vi "SliderAndBarTest.vi"(0 "Vertical Pointer Slide Control":dbl(slide) scale=0.0..10.0, 1 "Vertical Progress Bar Control":i32(slide) scale=0.0..100.0, 2 "Vertical Graduated Bar Control":u8(slide) scale=0.0..100.0, 3 "Horizontal Fill Slide Control":dbl(slide) scale=0.0..10.0, 4 "Horizontal Pointer Slide Control":dbl(slide) scale=0.0..10.0, 5 "Horizontal Progress Bar Control":u8(slide) scale=0.0..100.0, 6 "Vertical Fill Slide Control":dbl(slide) scale=0.0..10.0, 7 "Horizontal Graduated Bar Control":u8(slide) scale=0.0..100.0, 8 "Number To Add With":i32) -> (12 "Vertical Fill Slide Indicator":dbl(slide) scale=0.0..10.0, 13 "Horizontal Graduated Bar Indicator":u8(slide) scale=0.0..100.0, 14 "Vertical Pointer Slide Indicator":dbl(slide) scale=0.0..10.0, 15 "Vertical Progress Bar Indicator":i32(slide) scale=0.0..100.0, 16 "Vertical Graduated Bar Indicator":u8(slide) scale=0.0..100.0, 17 "Horizontal Fill Slide Indicator":dbl(slide) scale=0.0..10.0, 18 "Horizontal Pointer Slide Indicator":dbl(slide) scale=0.0..10.0, 19 "Horizontal Progress Bar Indicator":u8(slide) scale=0.0..100.0)   [LabVIEW 2012]
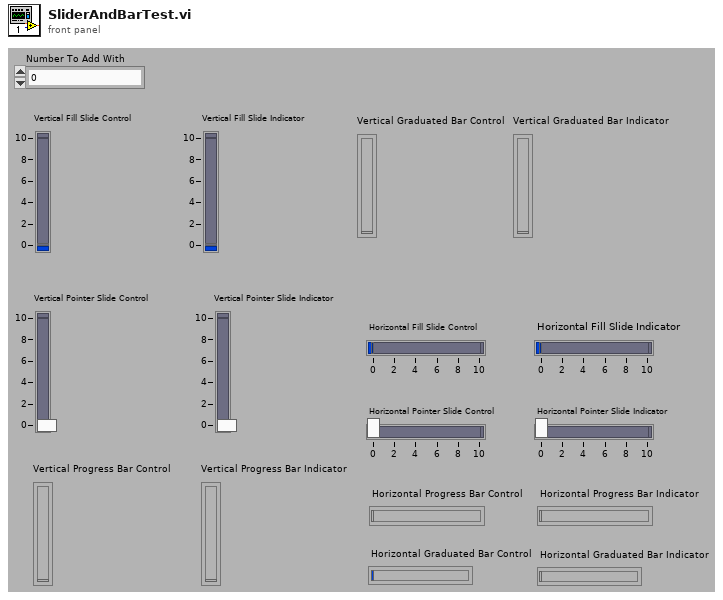
[diagram p1: front panel]
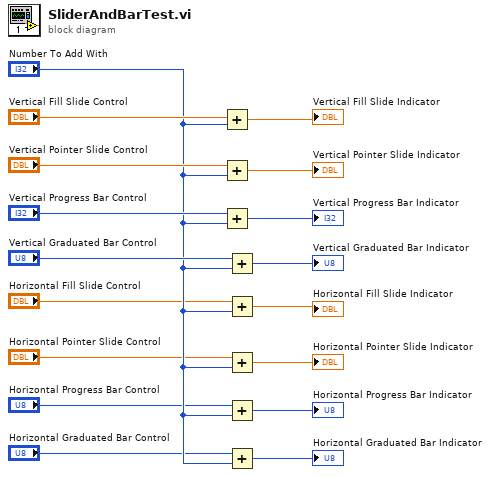
[diagram p0: block diagram]
diagram:
  n1 = Add(x="Vertical Fill Slide Control", y="Number To Add With") -> (x+y=→"Vertical Fill Slide Indicator":dbl)
  n2 = Add(x="Vertical Pointer Slide Control", y="Number To Add With") -> (x+y=→"Vertical Pointer Slide Indicator":dbl)
  n3 = Add(x="Vertical Progress Bar Control", y="Number To Add With") -> (x+y=→"Vertical Progress Bar Indicator":i32)
  n4 = Add(x="Vertical Graduated Bar Control", y="Number To Add With") -> (x+y=→"Vertical Graduated Bar Indicator":i32)
  n5 = Add(x="Horizontal Fill Slide Control", y="Number To Add With") -> (x+y=→"Horizontal Fill Slide Indicator":dbl)
  n6 = Add(x="Horizontal Pointer Slide Control", y="Number To Add With") -> (x+y=→"Horizontal Pointer Slide Indicator":dbl)
  n7 = Add(x="Horizontal Progress Bar Control", y="Number To Add With") -> (x+y=→"Horizontal Progress Bar Indicator":i32)
  n8 = Add(x="Horizontal Graduated Bar Control", y="Number To Add With") -> (x+y=→"Horizontal Graduated Bar Indicator":i32)
